vi "sv_Check for Block location.vi"(6 "AI block size":i32, 7 "write index":u32, 11 "indice computations in":T1) -> (3 "indice computations in":T1, 4 "write index - block size":u32)   [LabVIEW 2017, in "SoundVib_SweptSine.lvlib"]
uses:
  <vilib>/addons/Sound and Vibration/svt_Swept Sine/SoundVib_SweptSine.lvlib
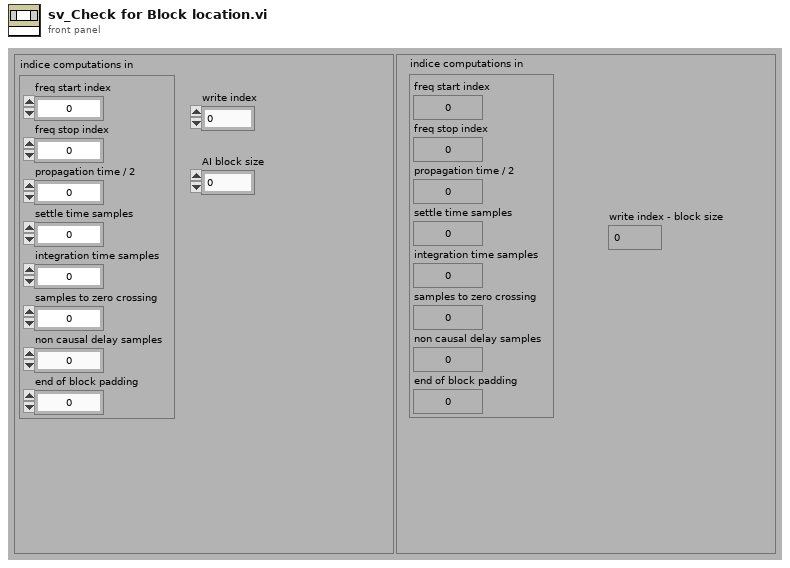
[diagram p1: front panel]
types:
  T1 = cluster{"freq start index":u32, "freq stop index":u32, "propagation time / 2":u32, "settle time samples":u32, "integration time samples":u32, "samples to zero crossing":u32, "non causal delay samples":u32, "end of block padding":u32}
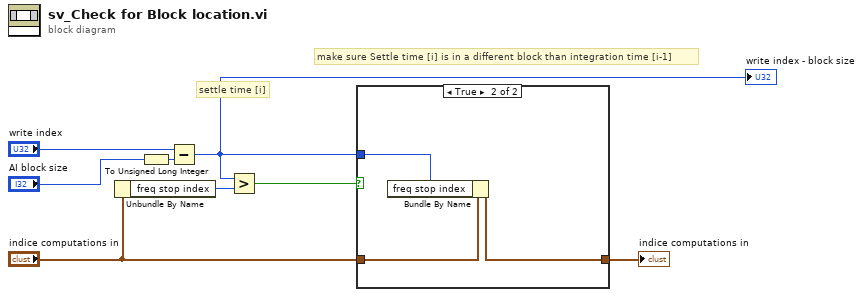
[diagram p0: block diagram]
diagram:
  # "make sure Settle time [i] is in a different block than integration time [i-1]"
  # "settle time [i]"
  n1 = Unbundle By Name("indice computations in") -> ("freq stop index"=w5:u32)
  n2 = To Unsigned Long Integer(number="AI block size") -> (unsigned 32bit integer=w1:u32)
  n3 = Subtract(x="write index", y=w1) -> (x-y=w4:u32)
  "write index - block size" <- w4
  n4 = Greater?(x=w4, y=w5) -> (0:w6:bool)
  n5 = case shown="True" w6 {
    tunnel: "indice computations in" -> [w9 w11]
    tunnel: [w9 w12] -> w7
    tunnel: w4 -> [_ w10]
    frame False {
      # "Settle time [i] is in a different buffer than \nIntegration time [i-1]"
    }
    frame True {
      n6 = Bundle By Name(cluster=w11, "freq stop index"=w10) -> (w12:T1)
    }
  }
  "indice computations in" <- w7
